vi "EditorThumbnail drawPicture.vi"(8 "error in (no error)":errorcluster, 11 "EditorThumbnail in":refnum<class "EditorThumbnail.lvclass">) -> (0 "error out":errorcluster, 3 "EditorThumbnail out":refnum<class "EditorThumbnail.lvclass">)   [LabVIEW 2018, in "EditorThumbnail.lvclass"]
uses:
  EditorThumbnail.lvclass
  <vilib>/Utility/miscctls.llb/LVBoundsTypeDef.ctl
  EditorThumbnail.lvclass/EditorThumbnail.ctl
panel:
  out "Temp":cluster{"X":dbl[], "Y":sgl[]}[](graph)
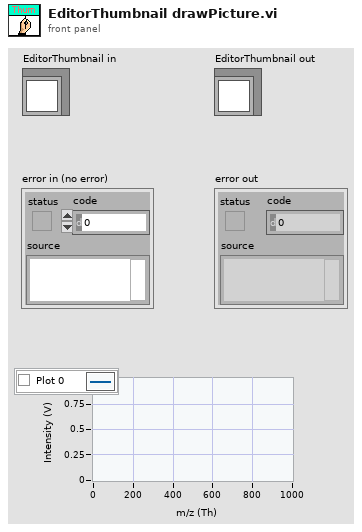
[diagram p1: front panel]
types:
  T1 = typedef "LVBoundsTypeDef.ctl" = cluster{"Width":u32, "Height":u32}
  T2 = cluster{"index":u32, "data":cluster{"xdata":dbl[], "ydata":sgl[]}[], "peak":dbl[], "picture":picture}[]
  T3 = typedef "imagedata.ctl" = cluster{"image type":i32, "image depth":i32, "image":u8[], "mask":u8[], "colors":u32[], "Rectangle":cluster{"left":i16, "top":i16, "right":i16, "bottom":i16}}
  T4 = cluster{"index":u32, "data":cluster{"xdata":dbl[], "ydata":sgl[]}[], "peak":dbl[], "picture":picture}
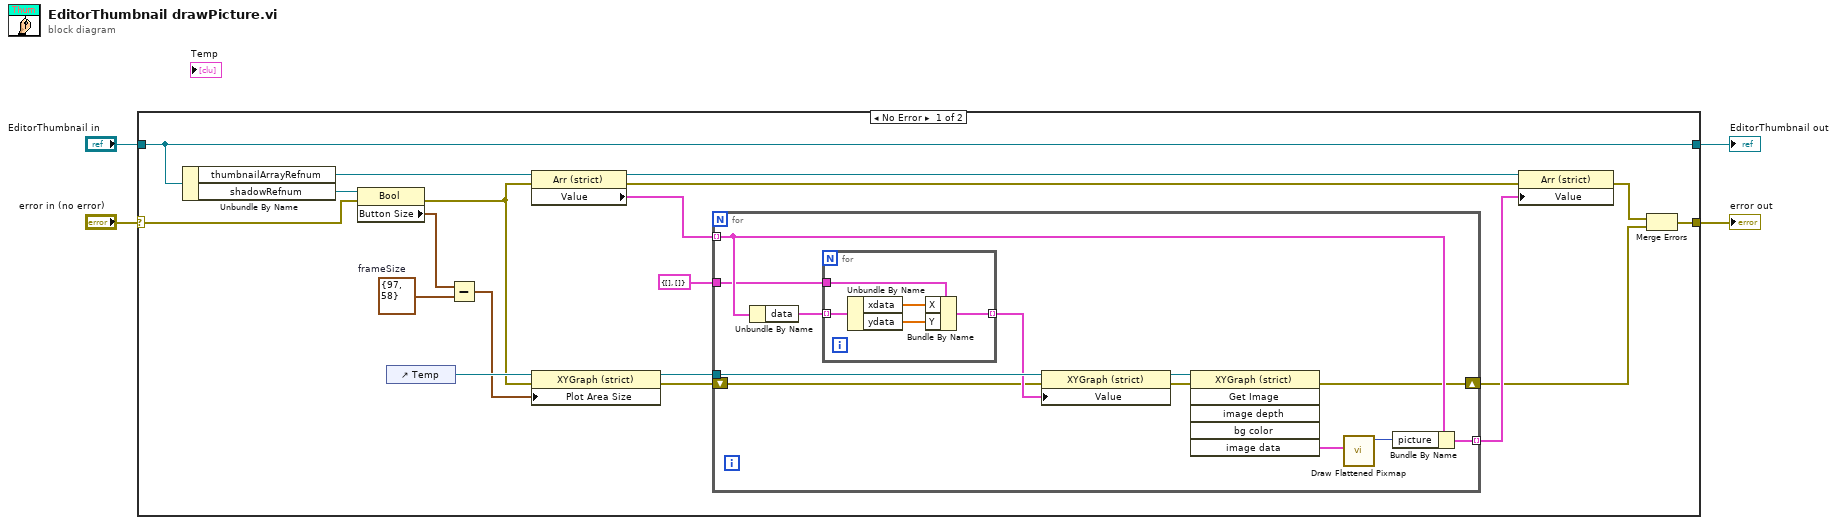
[diagram p0: block diagram]
diagram:
  n1 = case shown="No Error" "error in (no error)" {
    selector: "error in (no error)" -> [w11 w42]
    tunnel: [w6 w42] -> w3
    tunnel: [w23 w41] -> w1
    tunnel: "EditorThumbnail in" -> [w23 w41]
    frame No Error {
      w18 = T1 {"Width"=97, "Height"=58}  # frameSize
      n2 = Unbundle By Name(w23) -> ("thumbnailArrayRefnum"=w22:refnum<vi>, "shadowRefnum"=w20:refnum<vi>)
      n3 = property class="Bool"(reference=w20, error in=w11) -> (error out=w10:errorcluster, "Button Size"=w19:T1)  [unwired: 1 out]
      n4 = control-ref of="Temp"() -> (w17:refnum<vi>)
      n5 = Subtract(x=w19, y=w18) -> (x-y=w16:T1)
      n6 = property class="Arr (strict)"(reference=w22, error in=w10) -> (reference out=w13:refnum<vi>, error out=w9:errorcluster, "Value"=w21:T2)
      n7 = property class="XYGraph (strict)"(reference=w17, error in=w10, "Plot Area Size"=w16) -> (reference out=w15:refnum<vi>, error out=w8:errorcluster)
      n8 = for {
        tunnel: w21 -> [w29] mode=indexing
        tunnel: w15 -> [w34]
        tunnel: cluster{"X":dbl[], "Y":sgl[]} {"X"=[], "Y"=[]} ("Spectrum in") -> [w27]
        tunnel: [w26] -> w12 mode=indexing
        shift-right: [w24] -> w5
        shift-left: w8 -> [w25]
        n9 = Unbundle By Name(w29) -> ("data"=w35:cluster{"xdata":dbl[], "ydata":sgl[]}[])
        n10 = for {
          tunnel: w35 -> [w40] mode=indexing
          tunnel: [w37] -> w33 mode=indexing
          tunnel: w27 -> [w36]
          n11 = Unbundle By Name(w40) -> ("xdata"=w39:dbl[], "ydata"=w38:sgl[])
          n12 = Bundle By Name(cluster=w36, "X"=w39, "Y"=w38) -> (w37:cluster{"X":dbl[], "Y":sgl[]})
        }
        n13 = property class="XYGraph (strict)"(reference=w34, error in=w25, "Value"=w33) -> (reference out=w32:refnum<vi>, error out=w31:errorcluster)
        n14 = invoke class="XYGraph (strict)" method="Get Image"(reference=w32, error in=w31) -> (error out=w24:errorcluster, "image data"=w30:T3)  [unwired: 4 in, 4 out]
        n15 = call <vilib>:"Draw Flattened Pixmap.vi"("image data"=w30) -> ("new picture"=w28:picture)  [unwired: 8 in]
        n16 = Bundle By Name(cluster=w29, "picture"=w28) -> (w26:T4)
      }
      n17 = property class="Arr (strict)"(reference=w13, error in=w9, "Value"=w12) -> (error out=w7:errorcluster)  [unwired: 1 out]
      n18 = Merge Errors(w7, w5) -> (w6:errorcluster)
    }
    frame Error {
    }
  }
  "error out" <- w3
  "EditorThumbnail out" <- w1
